vi "collectSurveys.vi"() -> ()   [LabVIEW 2016]
panel:
  in  "Stave Name":string="Stave8"
  out "Python standard output":string
  out "Python Standard error":string
  in  "Working Directory to Python scripts":path
  in  "Folder to Module txt files":path
  # "Please try to keep it one word\ni.e. please don't use spaces"
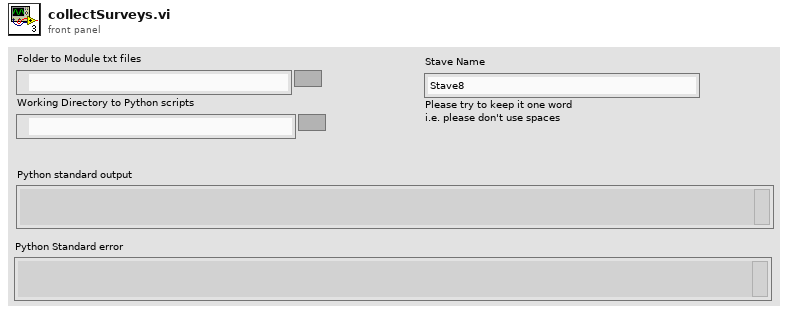
[diagram p1: front panel]
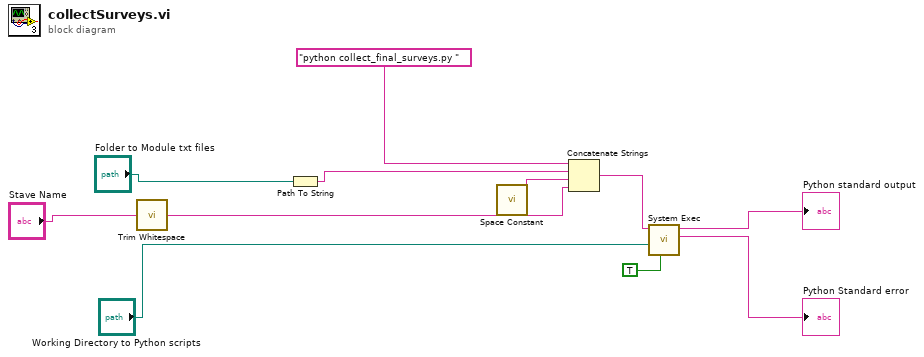
[diagram p0: block diagram]
diagram:
  n1 = call <vilib>:"Trim Whitespace.vi"("string"="Stave Name") -> ("trimmed string"=w1:string)  [unwired: 1 in]
  n2 = Path To String(path="Folder to Module txt files") -> (string=w8:string)
  n3 = call <vilib>:"Space Constant.vi"() -> ("String"=w2:string)
  n4 = Concatenate Strings("python collect_final_surveys.py ", w8, w2, w1) -> (w6:string)
  n5 = call <vilib>:"System Exec.vi"("run minimized? (F)"=TRUE, "working directory"="Working Directory to Python scripts", "command line"=w6) -> ("standard error"=→"Python Standard error":string, "standard output"=→"Python standard output":string)  [unwired: 5 in, 2 out]
